vi "save channels to separate multi-tiff files.vi"(8 "frame number in":i32, 9 "last frame":bool, 11 "image data in":dbl[][](array[numeric])) -> ()   [LabVIEW 2012]
uses:
  Custom Controls/file format type def.ctl
  GFG/GFGpathGet.vi
  GFG/GFGnumericGet.vi
  Libtiff3/libtiff3.llb/libtiff3.lvlib
  GFG/GFG library.lvlib
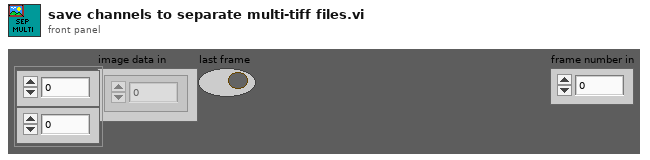
[diagram p1: front panel]
types:
  T1 = typedef "file format type def.ctl" = enum16{"16bit raw", "32bit raw", "16bit multi-tiff (interleave)", "16bit multi-tiff (separate)", "16bit multi-tiff (stacked)", "32bit multi-tiff (interleave)", "32bit multi-tiff (separate)", "32bit multi-tiff (stacked)", "16bit tiff series (interleave)", "16bit tiff series (separate)", "16bit tiff series (stacked)", "32bit tiff series (interleave)", "32bit tiff series (separate)", "32bit tiff series (stacked)"}
  T2 = cluster{"no..of.frames.to.acquire":dbl, "x.pixels":dbl, "y.pixels":dbl, "x.pixel.sz":dbl, "y.pixel.sz":dbl}
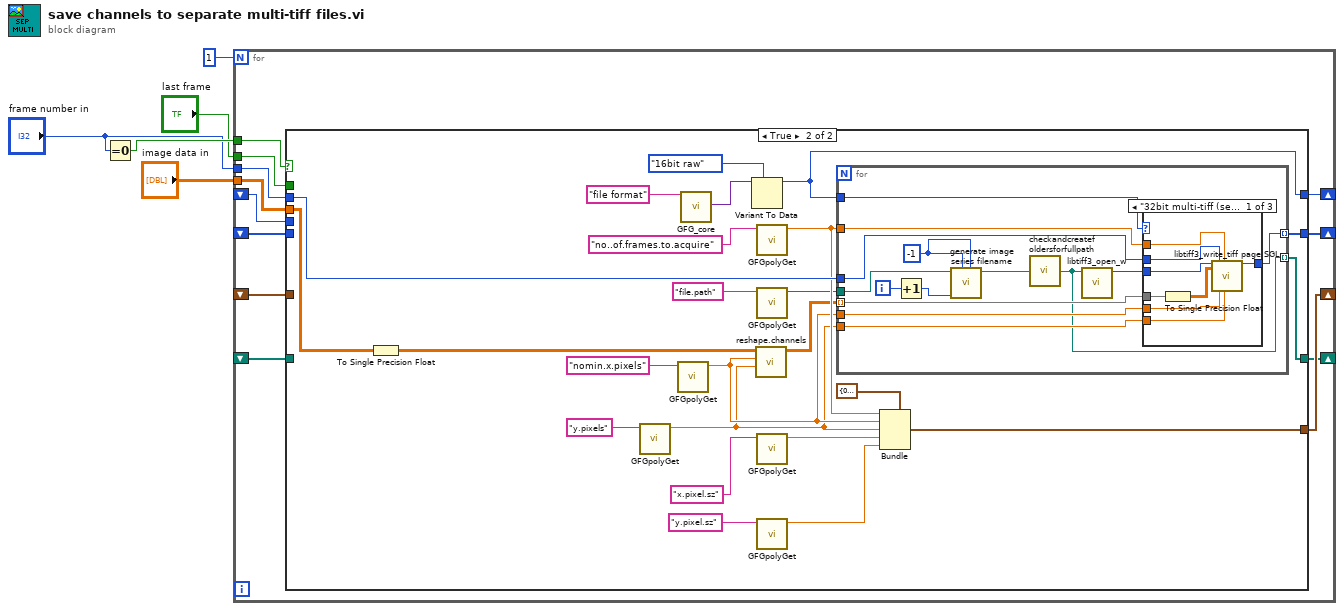
[diagram p0: block diagram]
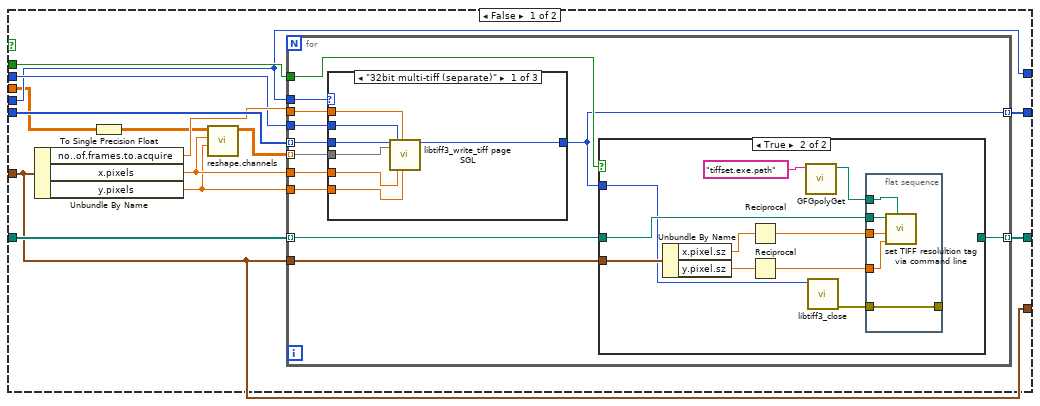
[diagram p2: hidden frame]
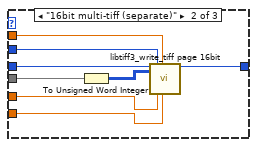
[diagram p3: hidden frame]
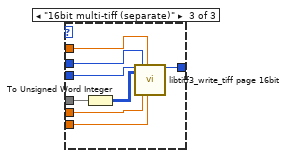
[diagram p7: hidden frame]
diagram:
  n1 = Equal To 0?(x="frame number in") -> (x = 0?=w4:bool)
  n2 = for {
    N: 1 -> [_]
    tunnel: w4 -> [w17]
    shift-right: [w16] -> _
    shift-left: _ -> [w15]
    tunnel: "image data in" -> [w14]
    shift-right: [w13] -> _
    shift-left: _ -> [w12]
    shift-right: [w11] -> _
    shift-left: _ -> [w10]
    shift-right: [w9] -> _
    shift-left: _ -> [w8]
    tunnel: "last frame" -> [w7]
    tunnel: "frame number in" -> [w6]
    n3 = case shown="True" w17 {
      tunnel: w12 -> [w25 _]
      tunnel: [w23 w83] -> w16
      tunnel: w15 -> [w29 _]
      tunnel: w14 -> [w22 w79]
      tunnel: [w25 w86] -> w13
      tunnel: [w24 w87] -> w11
      tunnel: w10 -> [w24 _]
      tunnel: [w28 w76] -> w9
      tunnel: w8 -> [w30 _]
      tunnel: w7 -> [w31 _]
      tunnel: w6 -> [w26 w85]
      frame False {
        n4 = Unbundle By Name(w24) -> ("no..of.frames.to.acquire"=w27:dbl, "x.pixels"=w19:dbl, "y.pixels"=w18:dbl)
        n5 = To Single Precision Float(number=w22) -> (single precision float=w21:sgl[][])
        n6 = call "reshape.channels.vi"("y.pixels"=w18, "x.pixels"=w19, "element"=w21) -> ("Array"=w20:dbl[][][])  [unwired: 8 in]
        n7 = for {
          tunnel: w31 -> [w43]
          tunnel: w30 -> [w42] mode=indexing
          tunnel: w20 -> [w41] mode=indexing
          tunnel: w29 -> [w40] mode=indexing
          tunnel: [w39] -> w28 mode=indexing
          tunnel: w27 -> [w38]
          tunnel: w26 -> [w37]
          tunnel: w19 -> [w36]
          tunnel: w18 -> [w35]
          tunnel: w25 -> [w34]
          tunnel: w24 -> [w33]
          tunnel: [w32] -> w23 mode=indexing
          n8 = case shown="\"32bit multi-tiff (separate)\"" w34 {
            tunnel: w41 -> [w44 w58 _]
            tunnel: w40 -> [w50 w56 w59]
            tunnel: [w47 w55 w59] -> w32
            tunnel: w38 -> [w48 w54 _]
            tunnel: w37 -> [w49 w53 _]
            tunnel: w36 -> [w46 w52 _]
            tunnel: w35 -> [w45 w51 _]
            frame "32bit multi-tiff (separate)" {
              n9 = call "libtiff3_write_tiff page SGL.vi"("Handle"=w50, "Image Pixels (Float)"=w44, "page"=w49, "x.pixels"=w46, "totalpages"=w48, "y.pixels"=w45) -> ("Handle out"=w47:i32)  [unwired: 12 in, 1 out]
            }
            frame "16bit multi-tiff (separate)" {
              n10 = To Unsigned Word Integer(number=w58) -> (unsigned 16bit integer=w57:u16[][])
              n11 = call "libtiff3_write_tiff page 16bit.vi"("Handle"=w56, "Image Pixels (U16)"=w57, "page"=w53, "x.pixels"=w52, "totalpages"=w54, "y.pixels"=w51) -> ("Handle out"=w55:i32)  [unwired: 12 in, 1 out]
            }
            frame Default {
            }
          }
          n12 = case shown="True" w43 {
            tunnel: w33 -> [_ w65]
            tunnel: w42 -> [w60 w64]
            tunnel: w32 -> [_ w63]
            tunnel: [w60 _] -> w39
            frame False {
            }
            frame True {
              n13 = Unbundle By Name(w65) -> ("x.pixel.sz"=w66:dbl, "y.pixel.sz"=w67:dbl)
              n14 = Reciprocal(x=w66) -> (1/x=w68:dbl)
              n15 = Reciprocal(x=w67) -> (1/x=w69:dbl)
              n16 = call-poly "GFGpolyGet.vi"("Variable Name in"="tiffset.exe.path") -> ("Path"=w61:path)  [unwired: 9 in, 1 out]
              n17 = call "libtiff3_close.vi"("Handle"=w63) -> ("error out"=w70:errorcluster)  [unwired: 9 in]
              n18 = flat-sequence {
                tunnel: w64 -> [w75]
                tunnel: w70 -> [w72]
                tunnel: w68 -> [w74]
                tunnel: w69 -> [w73]
                tunnel: [w72] -> _
                tunnel: w61 -> [w71]
                frame #0 {
                  n19 = call "set TIFF resolultion tag via command line.vi"("tiffset.exe file path"=w71, "y pixels per m"=w73, "x pixels per m"=w74, "TIFF file path"=w75) -> ()  [unwired: 8 in]
                }
              }
            }
          }
        }
      }
      frame True {
        n20 = To Single Precision Float(number=w79) -> (single precision float=w82:sgl[][])
        n21 = call-poly "GFGpolyGet.vi"("Variable Name in"="y.pixels" ("Tag in")) -> ("Numeric"=w80:dbl)  [unwired: 9 in, 1 out]
        n22 = call-poly "GFGpolyGet.vi"("Variable Name in"="nomin.x.pixels" ("Tag in")) -> ("Numeric"=w81:dbl)  [unwired: 9 in, 1 out]
        n23 = call "GFG_core.vi"("Variable Name in"="file format") -> ("Variant Out"=w98:variant)  [unwired: 12 in, 6 out]
        n24 = Variant To Data(type=file_format_type_def."16bit raw" ("file format"), Variant=w98) -> (data=w86:T1)  [unwired: 1 in, 1 out]
        n25 = call "reshape.channels.vi"("y.pixels"=w80, "x.pixels"=w81, "element"=w82) -> ("Array"=w78:dbl[][][])  [unwired: 8 in]
        n26 = call-poly "GFGpolyGet.vi"("Variable Name in"="no..of.frames.to.acquire") -> ("Numeric"=w84:dbl)  [unwired: 9 in, 1 out]
        n27 = call-poly "GFGpolyGet.vi"("Variable Name in"="file.path") -> ("Path"=w77:path)  [unwired: 9 in, 1 out]
        n28 = call-poly "GFGpolyGet.vi"("Variable Name in"="x.pixel.sz" ("Tag in")) -> ("Numeric"=w90:dbl)  [unwired: 9 in, 1 out]
        n29 = call-poly "GFGpolyGet.vi"("Variable Name in"="y.pixel.sz" ("Tag in")) -> ("Numeric"=w89:dbl)  [unwired: 9 in, 1 out]
        n30 = for {
          tunnel: w86 -> [w113]
          tunnel: w85 -> [w112]
          tunnel: w84 -> [w111]
          tunnel: [w110] -> w83 mode=indexing
          tunnel: w81 -> [w109]
          tunnel: w80 -> [w108]
          tunnel: w78 -> [w107] mode=indexing
          tunnel: w77 -> [w103]
          tunnel: [w100] -> w76 mode=indexing
          i -> [w105]
          w102 = -1 ("frame number in")
          n31 = Increment(x=w105) -> (x+1=w104:i32)
          n32 = call "generate image series filename.vi"("frame number in"=w102, "no..of.frames.to.acquire"=w102, "channel"=w104, "Path IN"=w103) -> ("appended path"=w101:path)  [unwired: 7 in]
          n33 = call "checkandcreatefoldersforfullpath.vi"("Path IN"=w101) -> ("Path OUT"=w100:path)  [unwired: 4 in]
          n34 = call "libtiff3_open_w.vi"("Input path"=w100) -> ("handle"=w106:i32)  [unwired: 9 in, 1 out]
          n35 = case shown="\"32bit multi-tiff (separate)\"" w113 {
            tunnel: w107 -> [w117 _ w127]
            tunnel: w106 -> [w118 w122 w128]
            tunnel: w112 -> [w119 _ w129]
            tunnel: w111 -> [w120 _ w130]
            tunnel: [w121 w122 w123] -> w110
            tunnel: w109 -> [w114 _ w125]
            tunnel: w108 -> [w115 _ w124]
            frame "32bit multi-tiff (separate)" {
              n36 = To Single Precision Float(number=w117) -> (single precision float=w116:sgl[][])
              n37 = call "libtiff3_write_tiff page SGL.vi"("Handle"=w118, "Image Pixels (Float)"=w116, "page"=w119, "x.pixels"=w114, "totalpages"=w120, "y.pixels"=w115) -> ("Handle out"=w121:i32)  [unwired: 12 in, 1 out]
            }
            frame Default {
            }
            frame "16bit multi-tiff (separate)" {
              n38 = To Unsigned Word Integer(number=w127) -> (unsigned 16bit integer=w126:u16[][])
              n39 = call "libtiff3_write_tiff page 16bit.vi"("Handle"=w128, "Image Pixels (U16)"=w126, "page"=w129, "x.pixels"=w125, "totalpages"=w130, "y.pixels"=w124) -> ("Handle out"=w123:i32)  [unwired: 12 in, 1 out]
            }
          }
        }
        n40 = Bundle(cluster=T2 {"no..of.frames.to.acquire"=0.0, "x.pixels"=0.0, "y.pixels"=0.0, "x.pixel.sz"=0.0, "y.pixel.sz"=0.0} ("output cluster"), "no..of.frames.to.acquire"=w84, "x.pixels"=w81, "y.pixels"=w80, "x.pixel.sz"=w90, "y.pixel.sz"=w89) -> (w87:T2)
      }
    }
  }
